vi "Write JSON Config.vi"(6 "Pretty Print?":bool, 8 "error in (no error)":errorcluster, 11 "AbsComp_Two Term_STR in":refnum<class "AbsComp_Two Term_STR.lvclass">) -> (0 "error out":errorcluster, 2 "JSON":string, 3 "AbsComp_Two Term_STR out":refnum<class "AbsComp_Two Term_STR.lvclass">)   [LabVIEW 2021, in "AbsComp_Two Term_STR.lvclass"]
uses:
  AbsComp_Two Term_STR.lvclass
  C:/Program Files (x86)/National Instruments/LabVIEW 2021/vi.lib/TSA/Abstract Data Classes/Abs_Types/Type/Abs_Type.lvclass
  AbsComp_Two Term_STR.lvclass/AbsComp_Two Term_STR.ctl
  <vilib>/JDP Science/JSONtext/Make JSON Array.vi
  <vilib>/JDP Science/JSONtext/Merge into Object.vi
  <vilib>/JDP Science/JSONtext/Make JSON Object.vi
  <vilib>/Utility/LVClass/Get LV Class Name.vi
  <vilib>/JDP Science/JSONtext/support/Format JSON Array Text.vi
  <vilib>/JDP Science/JSONtext/support/Format JSON Object.vi
  <vilib>/JDP Science/JSONtext/Get all Object Items.vi
  <vilib>/JDP Science/JSONtext/Set Multiple Object Items.vi
  Abs_Types/String/Abs_String.lvclass
  Abs_Types/Boolean/Abs_Boolean.lvclass
  Abs_Types/Type/Abs_Type.lvclass
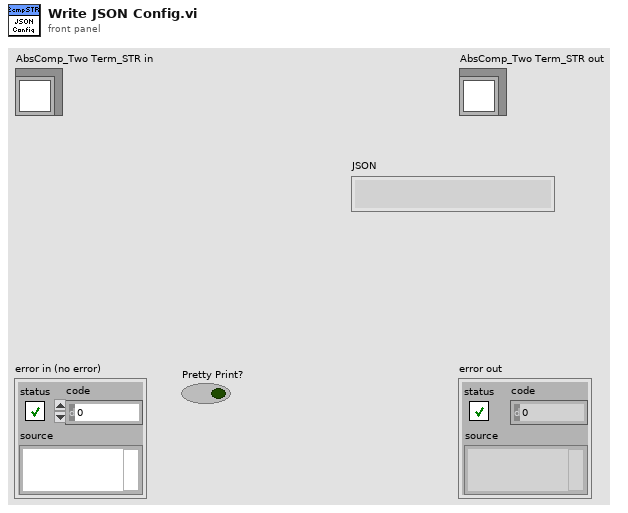
[diagram p1: front panel]
types:
  T1 = typedef "AbsComp_Two Term_STR.lvclass/Abstract Type.ctl" = refnum<class "Abs_String.lvclass">
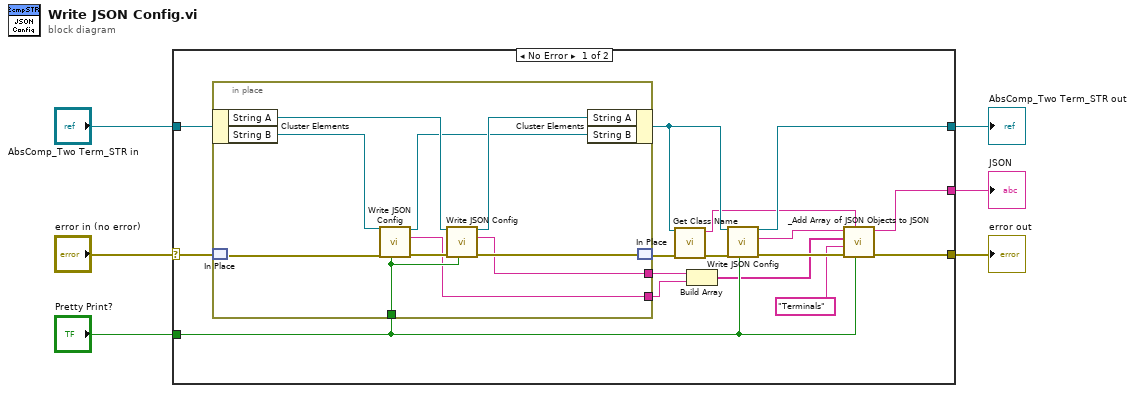
[diagram p0: block diagram]
diagram:
  n1 = case shown="No Error" "error in (no error)" {
    selector: "error in (no error)" -> [w17 w34]
    tunnel: "AbsComp_Two Term_STR in" -> [w22 w33]
    tunnel: [w21 w33] -> w1
    tunnel: [w13 _] -> w2
    tunnel: [w12 w34] -> w3
    tunnel: "Pretty Print?" -> [w11 _]
    frame No Error {
      n2 = in-place {
        in-place-border: w11 -> [w30]
        in-place-border: [w28] -> w20
        in-place-border: [w27] -> w19
        n3 = in-place-cluster #1(w22) -> ("String A"=w26:T1, "String B"=w24:refnum<class "Abs_String.lvclass">)
        n4 = in-place-match #2(w17) -> (w31:errorcluster)
        n5 = call-dynamic "Write JSON Config.vi"("Pretty Print?"=w30, "error in (no error)"=w31, "Abs_Type in"=w24) -> ("error out"=w32:errorcluster, "JSON"=w27:string, "Abs_Type out"=w23:refnum<class "Abs_String.lvclass">)  [unwired: 6 in]
        n6 = call-dynamic "Write JSON Config.vi"("Pretty Print?"=w30, "error in (no error)"=w32, "Abs_Type in"=w26) -> ("error out"=w29:errorcluster, "JSON"=w28:string, "Abs_Type out"=w25:T1)  [unwired: 6 in]
        n7 = in-place-cluster #1("String A"=w25, "String B"=w23) -> (w15:refnum<class "AbsComp_Two Term_STR.lvclass">)
        n8 = in-place-match #2(w29) -> (w18:errorcluster)
      }
      n9 = call "Get Class Name.vi"("error in (no error)"=w18, "Abs_Type in"=w15) -> ("error out"=w16:errorcluster, "class name"=w10:string)  [unwired: 8 in]
      n10 = Build Array(w20, w19) -> (w8:string[])
      n11 = call-parent "Write JSON Config.vi"("Pretty Print?"=w11, "error in (no error)"=w16, "Abs_Type in"=w15) -> ("error out"=w14:errorcluster, "JSON"=w9:string, "Abs_Type out"=w21:refnum<class "AbsComp_Two Term_STR.lvclass">)  [unwired: 6 in]
      n12 = call "_Add Array of JSON Objects to JSON.vi"("Pretty Print?"=w11, "JSON Object Name"=w10, "error in (no error)"=w14, "JSON Array Name"="Terminals", "JSON Objects"=w8, "JSON"=w9) -> ("error out"=w12:errorcluster, "<JSON>"=w13:string)  [unwired: 4 in]
    }
    frame Error {
    }
  }
  "error out" <- w3
  "AbsComp_Two Term_STR out" <- w1
  "JSON" <- w2
